vi "generate 1 cycle.vi"(8 "error in (no error)":errorcluster caption="에러 입력(에러 없음)", 11 "Auto Tracking Wave 입력":refnum<class "Auto Brake (Sine) Wave.lvclass">) -> (0 "error out":errorcluster caption="에러 출력", 2 "waveform":waveform(dbl), 3 "Auto Tracking Wave 출력":refnum<class "Auto Brake (Sine) Wave.lvclass">)   [LabVIEW 2020, in "Auto Brake (Sine) Wave.lvclass"]
uses:
  Auto Brake (Sine) Wave.lvclass
  Sine Wave/Sine Wave.lvclass
  Waveform Obj/Waveform Obj.lvclass/Waveform Obj.ctl
  Waveform Gen/Waveform Gen.lvclass/Waveform Gen.ctl
  Waveform Obj/Accessors/Read name.vi
  Waveform Obj/Accessors/Read sampling rate.vi
  Waveform Obj/Accessors/Read voltage range.vi
  Waveform Obj/Accessors/Read wait.vi
  Waveform Gen/Accessors/Read cycle.vi
  Waveform Gen/Accessors/Read offset.vi
  Waveform Gen/Accessors/Read phase.vi
  Waveform Gen/Accessors/Read repeat type.vi
  Waveform Gen/Accessors/Read scale.vi
  Waveform Obj/Accessors/Write name.vi
  Waveform Obj/Accessors/Write sampling rate.vi
  Waveform Obj/Accessors/Write voltage range.vi
  Waveform Obj/Accessors/Write wait.vi
  Waveform Gen/Accessors/Write offset.vi
  Waveform Gen/Accessors/Write phase.vi
  Waveform Gen/Accessors/Write repeat type.vi
  Waveform Gen/Accessors/Write scale.vi
  Waveform Gen/Accessors/Write frequency.vi
  Waveform Gen/Waveform Gen.lvclass
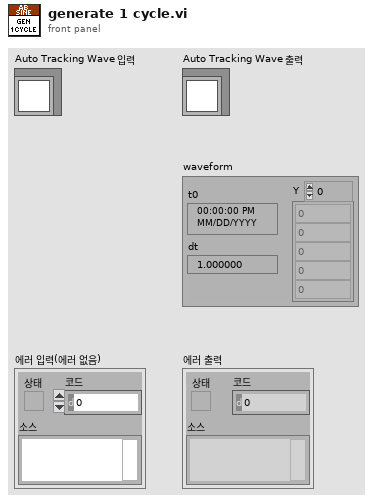
[diagram p1: front panel]
types:
  T1 = typedef "Waveform Gen.lvclass/repeat scale.ctl" = enum16{"Normal", "Lin. Up", "Lin. Down", "Exp. Up", "Exp. Down"}
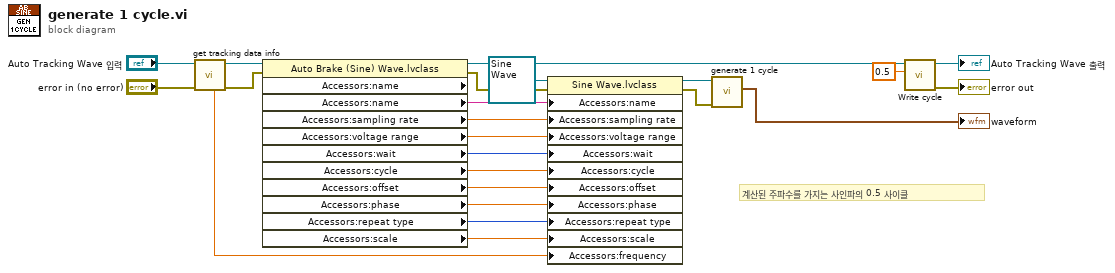
[diagram p0: block diagram]
diagram:
  # "계산된 주파수를 가지는 사인파의 0.5 사이클"
  n1 = call-dynamic "get tracking data info.vi"("error in (no error)"="error in (no error)", "Auto Tracking Wave 입력"="Auto Tracking Wave 입력") -> ("error out"=w7:errorcluster, "Auto Tracking Wave 출력"=w5:refnum<class "Auto Brake (Sine) Wave.lvclass">, "brake wave freq"=w4:dbl)  [unwired: 5 in, 2 out]
  n2 = property class="Auto Brake (Sine) Wave.lvclass" props=["Accessors:name", "Accessors:name", "Accessors:sampling rate", "Accessors:voltage range", "Accessors:wait", "Accessors:cycle", "Accessors:offset", "Accessors:phase", "Accessors:repeat type", "Accessors:scale"](reference=w5, error in=w7) -> (reference out=w2:refnum<class "Auto Brake (Sine) Wave.lvclass">, error out=w10:errorcluster, "Accessors:name"=w19:string, "Accessors:sampling rate"=w18:dbl, "Accessors:voltage range"=w17:dbl, "Accessors:wait"=w16:u8, "Accessors:cycle"=w15:dbl, "Accessors:offset"=w14:dbl, "Accessors:phase"=w13:dbl, "Accessors:repeat type"=w12:T1, "Accessors:scale"=w11:dbl)  [unwired: 1 out]
  n3 = property class="Sine Wave.lvclass"(reference=refnum<class "Sine Wave.lvclass"> refnum ("Sine Wave.lvclass"), error in=w10, "Accessors:name"=w19, "Accessors:sampling rate"=w18, "Accessors:voltage range"=w17, "Accessors:wait"=w16, "Accessors:cycle"=w15, "Accessors:offset"=w14, "Accessors:phase"=w13, "Accessors:repeat type"=w12, "Accessors:scale"=w11, "Accessors:frequency"=w4) -> (reference out=w8:refnum<class "Sine Wave.lvclass">, error out=w9:errorcluster)
  n4 = call-dynamic "generate 1 cycle.vi"("error in (no error)"=w9, "Sine Wave 입력"=w8) -> ("waveform"=→"waveform":waveform(dbl))  [unwired: 7 in, 2 out]
  n5 = call "Write cycle.vi"("cycle"=0.5, "Waveform Obj 입력"=w2) -> ("error out"=→"error out":errorcluster, "Waveform Obj 출력"=→"Auto Tracking Wave 출력":refnum<class "Auto Brake (Sine) Wave.lvclass">)  [unwired: 8 in]
